vi "tearDown.vi"(8 "error in (no error)":errorcluster, 11 "TestConfigurationFileBinding In":refnum<class "TestPersistToDiskTransport.lvclass">) -> (0 "error out":errorcluster, 3 "TestConfigurationFileBinding Out":refnum<class "TestPersistToDiskTransport.lvclass">)   [LabVIEW 2017, in "TestPersistToDiskTransport.lvclass"]
doc: "tearDown runs after the test method has completed. Use this method to clean up any operations or references that were opened by setUp or the test method. Unit tests should be independent of other unit tests so this VI should ensure that the next test can run in a 'clean' test environment."
uses:
  TestPersistToDiskTransport.lvclass
  TestPersistToDiskTransport.lvclass/TestPersistToDiskTransport.ctl
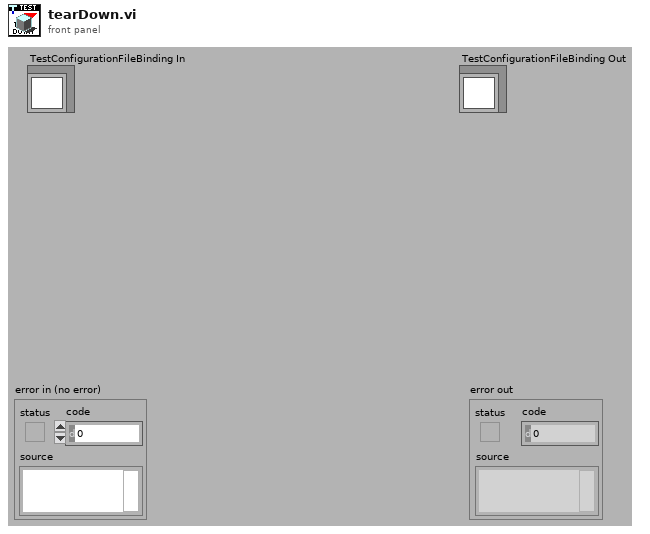
[diagram p1: front panel]
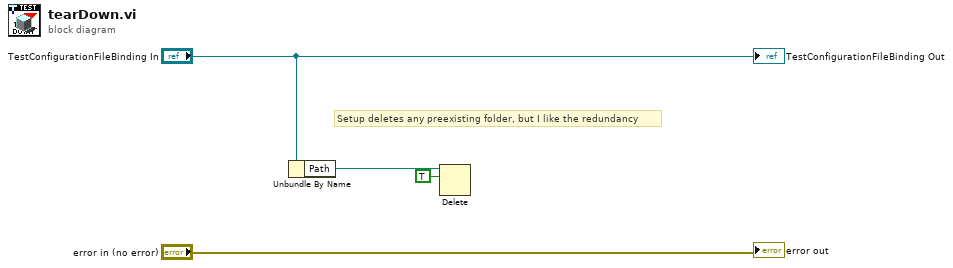
[diagram p0: block diagram]
diagram:
  # "Setup deletes any preexisting folder, but I like the redundancy"
  n1 = Unbundle By Name("TestConfigurationFileBinding In") -> ("Path"=w1:path)
  n2 = Delete(path (use dialog)=w1, entire hierarchy (F)=TRUE) -> ()  [unwired: 3 in, 3 out]
  "error out" <- "error in (no error)"
  "TestConfigurationFileBinding Out" <- "TestConfigurationFileBinding In"
